vi "PixyCam_SetBrightness.vi"(4 "error in (no error)":errorcluster, 6 "Brightness":u8, 7 "PixyCamDevRef":T1) -> (0 "error out":errorcluster, 3 "PixyCamDevRef Out":T1)   [LabVIEW 2016, in "PixyCam_LabVIEW.lvlib"]
uses:
  PixyCam_LabVIEW.lvlib
  Private/PixyCam_DevRef.ctl
  Private/PixyCam_SPI_DevRef.ctl
  <vilib>/Rock Robotics/WPI/SPI/WPI_SPIDevRef.ctl
  <vilib>/Rock Robotics/SystemInterfaces/spilib/spi_bus.ctl
  Private/PixyCam_CommMode.ctl
  Private/PixyCam_SerialByteConstants.ctl
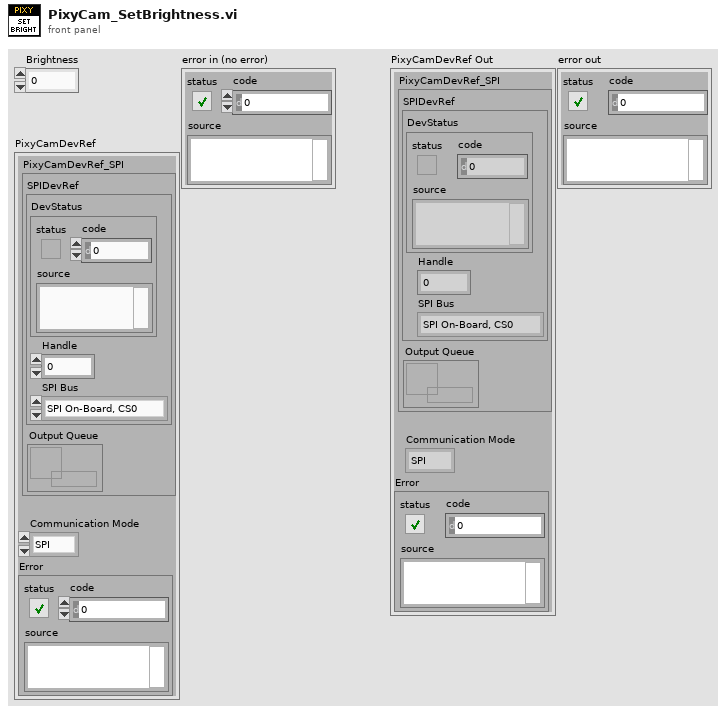
[diagram p1: front panel]
types:
  T1 = typedef "PixyCam_LabVIEW.lvlib/PixyCam_DevRef.ctl" = cluster{"PixyCamDevRef_SPI":T2, "Communication Mode":T5, "Error":errorcluster}
  T2 = typedef "PixyCam_LabVIEW.lvlib/PixyCam_SPI_DevRef.ctl" = cluster{"SPIDevRef":T3, "Output Queue":refnum<queue>}
  T3 = typedef "WPI_SPIDevRef.ctl" = cluster{"DevStatus":errorcluster, "Handle":i32, "SPI Bus":T4}
  T4 = typedef "spi_bus.ctl" = enum16{"SPI On-Board, CS0", "SPI On-Board, CS1", "SPI On-Board, CS2", "SPI On-Board, CS3", "SPI MXP", "Invalid"}
  T5 = typedef "PixyCam_LabVIEW.lvlib/PixyCam_CommMode.ctl" = enum16{"SPI", "I2C", "UART", "Analog", "Digital"}
  T6 = typedef "PixyCam_LabVIEW.lvlib/PixyCam_SerialByteConstants.ctl" = u8
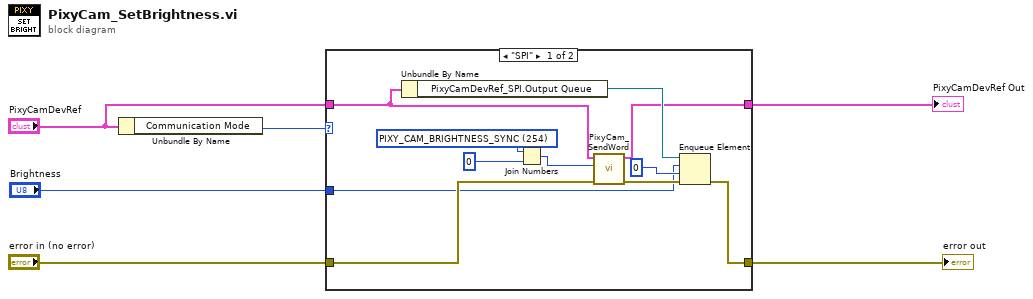
[diagram p0: block diagram]
diagram:
  n1 = Unbundle By Name("PixyCamDevRef") -> ("Communication Mode"=w6:T5)
  n2 = case shown="\"SPI\"" w6 {
    tunnel: "PixyCamDevRef" -> [w13 w19]
    tunnel: "error in (no error)" -> [w17 w18]
    tunnel: "Brightness" -> [w9 _]
    tunnel: [w8 w19] -> w2
    tunnel: [w7 w18] -> w1
    frame "SPI" {
      w16 = T6 254 items=["PIXY_SYNC_BYTE"=90, "PIXY_SYNC_BYTE_DATA"=91, "PIXY_SERVO_SYNC"=255, "PIXY_CAM_BRIGHTNESS_SYNC"=254, "PIXY_CAM_LED_SYNC"=253] ("SyncByte")
      n3 = Unbundle By Name(w13) -> ("PixyCamDevRef_SPI.Output Queue"=w12:refnum<queue>)
      n4 = Join Numbers(hi=w16, lo=u8 0 ("timeout in ms (-1)")) -> ((hi.lo)=w14:u16)
      n5 = call "PixyCam_SendWord.vi"("error in"=w17, "WriteWord"=w14, "PixyCamDevRef"=w13) -> ("error out"=w11:errorcluster, "PixyCamDevRef Out"=w8:T1)  [unwired: 3 in]
      n6 = Enqueue Element(queue=w12, element=w9, timeout in ms (-1)=0, error in (no error)=w11) -> (error out=w7:errorcluster)  [unwired: 2 out]
    }
    frame Default {
    }
  }
  "PixyCamDevRef Out" <- w2
  "error out" <- w1
